vi "RTI Connext DDS Write String.vi"() -> ()   [LabVIEW 2021]
doc: "Shows how to publish (write) a string using RTI Connext DDS. It was created using the simple read/write example in the Getting Started Guide (<LabVIEW folder>/help/RTI DDS Toolkit/RTI_DDS_Toolkit_GettingStarted.pdf)."
uses:
  <vilib>/RTI DDS Toolkit/VIs/SimpleCreateWriter_String.vi
  <vilib>/RTI DDS Toolkit/VIs/Write_String.vi
  <vilib>/RTI DDS Toolkit/VIs/Advanced Create Writer.vi
  <vilib>/RTI DDS Toolkit/VIs/AdvancedCreateWriter_String.vi
  <vilib>/RTI DDS Toolkit/Library/LVDDS_library.lvlib
panel:
  in  "Text":string
  in  "Stop Writing":bool
  in  "error in (no error)":errorcluster
  # "Overview: Demonstrate how to publish and write a String type using Connext DDS.\nRequirements: RTI DDS Toolkit\nInstructions:\n1. Run the VI.\n2. Run the RTI Connext DDS Read String.vi example.\n3. Modify the Text value and check whether the reader is receiving the correct information. \n\nMore information about this and other examples can be found in RTI_DDS_Toolkit_GettingStarted.pdf"
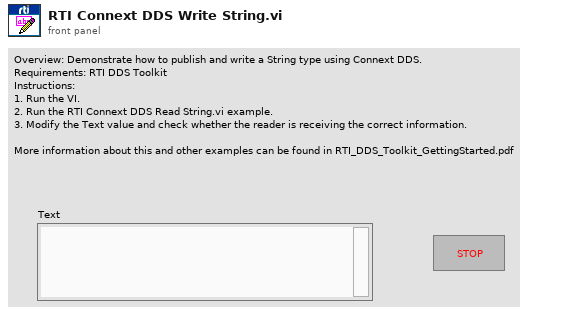
[diagram p1: front panel]
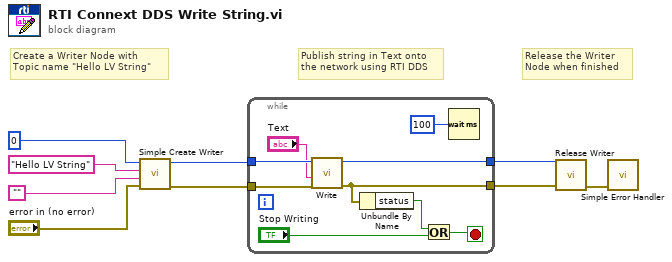
[diagram p0: block diagram]
diagram:
  # "Release the Writer \nNode when finished"
  # "Publish string in Text onto \nthe network using RTI DDS"
  # "Create a Writer Node with \nTopic name \"Hello LV String\""
  n1 = call-poly <vilib>:"Simple Create Writer.vi"("error in"="error in (no error)", "Type"="", "Topic Name"="Hello LV String", "Domain Id"=u32 0) -> ("error out"=w6:errorcluster, "DDS Object Ref"=w4:u64)  [unwired: 6 in]
  n2 = while {
    tunnel: w4 -> [w18]
    tunnel: [w17] -> w2
    tunnel: w6 -> [w16]
    tunnel: [w11] -> w3
    stop <- w13 stop-if-true
    n3 = call-poly <vilib>:"Write.vi"("error in (no error)"=w16, "Data"="Text", "DDS Object Ref in"=w18) -> ("error out"=w11:errorcluster, "DDS Object Ref out"=w17:u64)  [unwired: 7 in]
    n4 = Unbundle By Name(w11) -> ("status"=w14:bool)
    n5 = Or(x=w14, y="Stop Writing") -> (x .or. y?=w13:bool)
    n6 = Wait (ms)(milliseconds to wait=u32 100 ("millisecond multiple")) -> ()  [unwired: 1 out]
  }
  n7 = call <vilib>:"Release Writer.vi"("error in (no error)"=w3, "DDS Object Ref"=w2) -> ("error out"=w5:errorcluster)  [unwired: 9 in]
  n8 = call <vilib>:"Simple Error Handler.vi"("error in (no error)"=w5) -> ()  [unwired: 4 in, 5 out]
